vi "HW 3.vi"() -> ()   [LabVIEW 2020]
panel:
  in  "Quick Pick":bool
  out "Quick Picks":dbl[](array[numeric]) min=0.0 max=99.0 step=1.0
  in  "Done":bool
  in  "Play":bool
  out "Winnings":dbl
  out "Bank":dbl
  in  "Bet":dbl
  out "Results":dbl[](array[numeric]) min=0.0 max=99.0 step=1.0
  in  "Manual Picks":dbl[](array[numeric]) min=0.0 max=99.0 step=1.0
  # "Lucky 6"
  # "$"
  # "Toggle quick pick button on to use quick picks! When toggled off, the manual picks will be used to calculate the winnings."
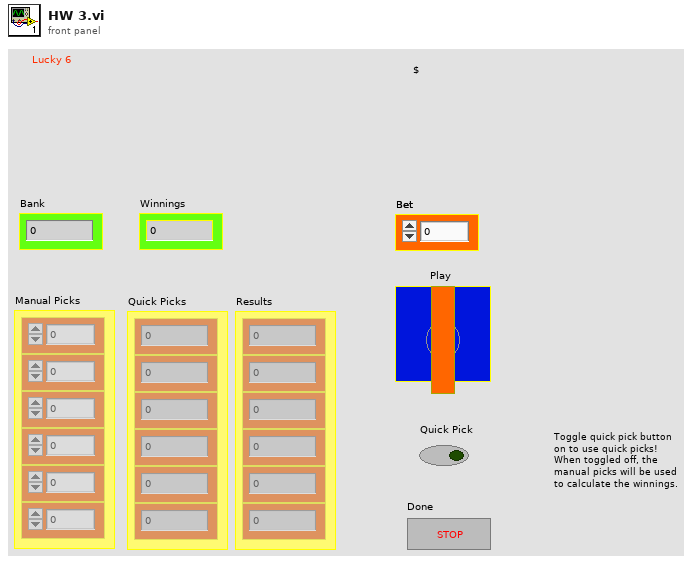
[diagram p1: front panel]
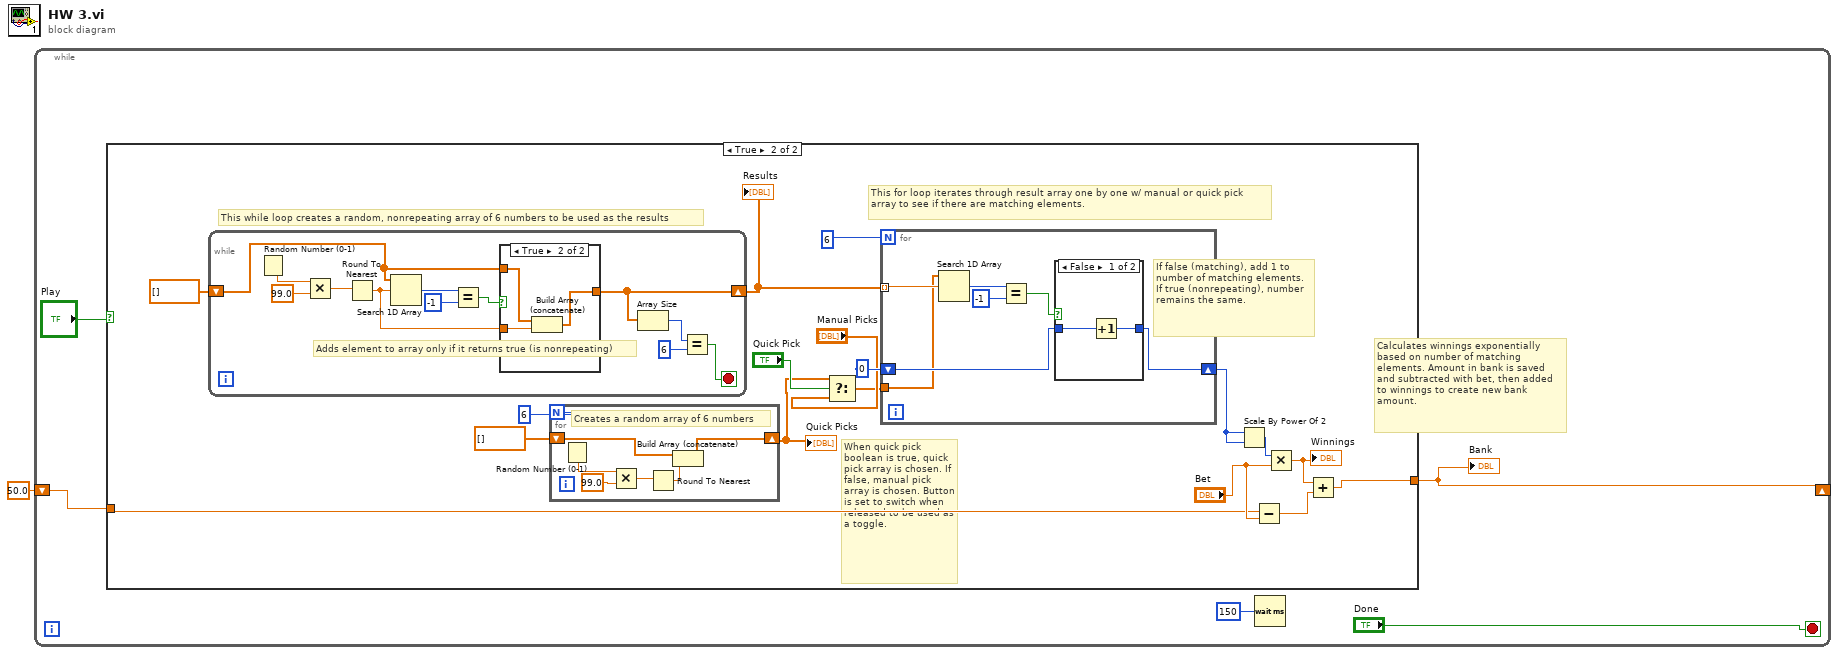
[diagram p0: block diagram]
diagram:
  n1 = while {
    shift-right: [w5] -> _
    shift-left: 50.0 -> [w4]
    stop <- "Done" stop-if-true
    # "Calculates winnings exponentially based on number of matching elements. Amount in bank is saved and subtracted with bet, then added to winnings to create new bank amount."
    n2 = case shown="True" "Play" {
      tunnel: [w7 w15] -> w5
      tunnel: w4 -> [w7 w14]
      frame False {
        # "On an iteration when the play button returns false, bank information is saved."
      }
      frame True {
        # "If false (matching), add 1 to number of matching elements. If true (nonrepeating), number remains the same."
        # "This for loop iterates through result array one by one w/ manual or quick pick array to see if there are matching elements."
        # "This while loop creates a random, nonrepeating array of 6 numbers to be used as the results"
        # "When quick pick boolean is true, quick pick array is chosen. If false, manual pick array is chosen. Button is set to switch when released to be used as a toggle."
        n3 = while {
          shift-right: [w44] -> w22
          shift-left: dbl[] [] -> [w45]
          stop <- w41 stop-if-true
          # "Adds element to array only if it returns true (is nonrepeating)"
          n4 = Random Number (0-1)() -> (number: 0 to 1=w52:dbl)
          n5 = Multiply(x=w52, y=99.0) -> (x*y=w50:dbl)
          n6 = Round To Nearest(number=w50) -> (nearest integer value=w46:dbl)
          n7 = Search 1D Array(1D array=w45, element=w46) -> (index of element=w49:i32)  [unwired: 1 in]
          n8 = Equal?(x=w49, y=-1) -> (x = y?=w47:bool)
          n9 = case shown="True" w47 {
            tunnel: w46 -> [_ w56]
            tunnel: [w53 w55] -> w44
            tunnel: w45 -> [w53 w54]
            frame False {
            }
            frame True {
              n10 = Build Array (concatenate)(w54, w56) -> (w55:dbl[])
            }
          }
          n11 = Array Size(array=w44) -> (size(s)=w43:i32)
          n12 = Equal?(x=w43, y=6) -> (x = y?=w41:bool)
        }
        "Results" <- w22
        n13 = for {
          N: 6 -> [_]
          shift-right: [w25] -> w9
          shift-left: dbl[] [] -> [w26]
          # "Creates a random array of 6 numbers"
          n14 = Random Number (0-1)() -> (number: 0 to 1=w29:dbl)
          n15 = Multiply(x=w29, y=99.0) -> (x*y=w30:dbl)
          n16 = Round To Nearest(number=w30) -> (nearest integer value=w27:dbl)
          n17 = Build Array (concatenate)(w26, w27) -> (w25:dbl[])
        }
        "Quick Picks" <- w9
        n18 = Select(t=w9, s="Quick Pick", f="Manual Picks") -> (s? t:f=w8:dbl[])
        n19 = for {
          N: 6 -> [_]
          tunnel: w22 -> [w35] mode=indexing
          shift-right: [w32] -> w20
          shift-left: 0 -> [w33]
          tunnel: w8 -> [w31]
          n20 = Search 1D Array(1D array=w31, element=w35) -> (index of element=w37:i32)  [unwired: 1 in]
          n21 = Equal?(x=w37, y=-1) -> (x = y?=w34:bool)
          n22 = case shown="False" w34 {
            tunnel: [w39 w40] -> w32
            tunnel: w33 -> [w38 w40]
            frame False {
              n23 = Increment(x=w38) -> (x+1=w39:i32)
            }
            frame True {
            }
          }
        }
        n24 = Scale By Power Of 2(n=w20, x=w20) -> (x*2^n=w19:i32)
        n25 = Subtract(x=w14, y="Bet") -> (x-y=w18:dbl)
        n26 = Multiply(x=w19, y="Bet") -> (x*y=w17:dbl)
        "Winnings" <- w17
        n27 = Add(x=w17, y=w18) -> (x+y=w15:dbl)
      }
    }
    "Bank" <- w5
    n28 = Wait (ms)(milliseconds to wait=u32 150) -> ()  [unwired: 1 out]
  }
